vi "basic_subvi_and or search.vi"(6 "key words":string, 7 "String array input":string[](array[string])) -> (0 "or condition key words":string[](array[string]), 1 "and condition key words":string[](array[string]), 2 "index of string w/ key words":i32[](array[numeric]), 3 "output string array w/ key words":string[](array[string]))   [LabVIEW 2020, in "BasicVIs.lvlib"]
uses:
  BasicVIs.lvlib
panel:
  out "finished whole string?":bool
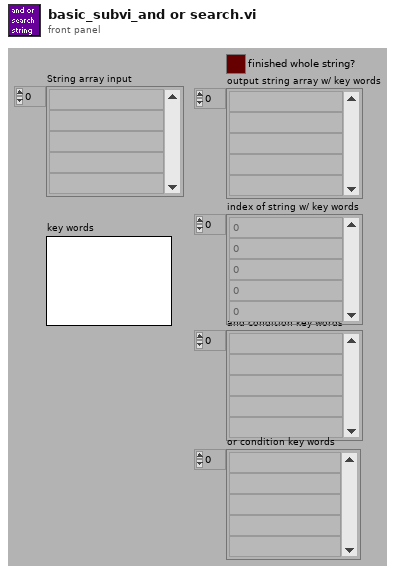
[diagram p1: front panel]
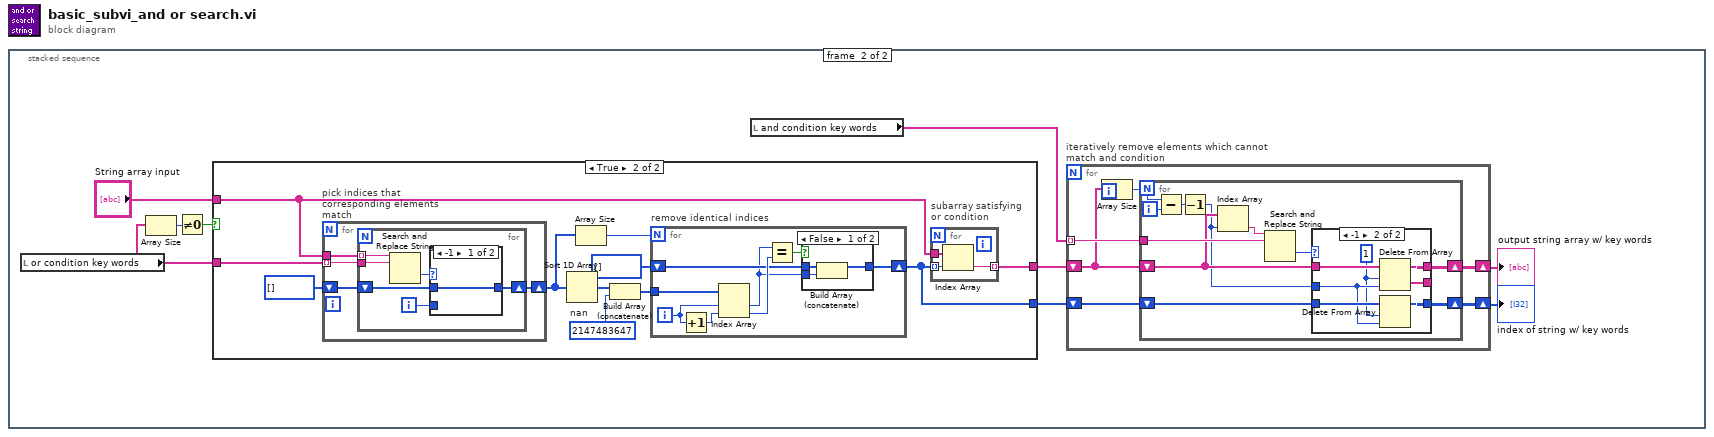
[diagram p0: block diagram]
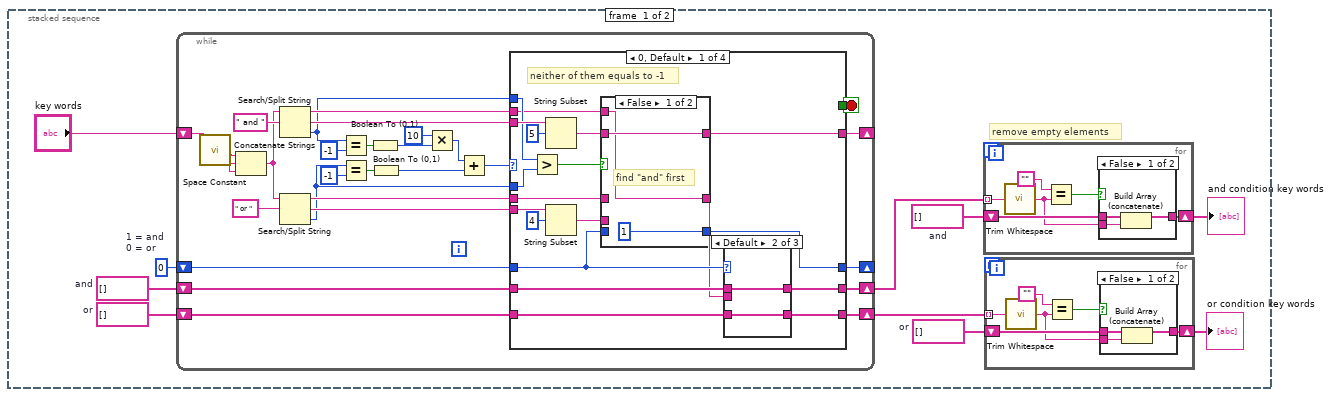
[diagram p2: hidden frame]
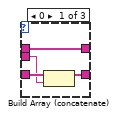
[diagram p5: hidden frame]
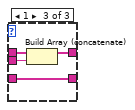
[diagram p6: hidden frame]
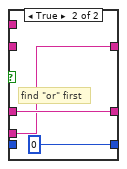
[diagram p7: hidden frame]
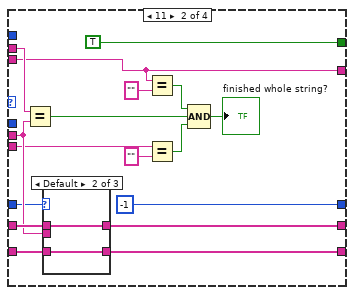
[diagram p8: hidden frame]
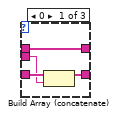
[diagram p9: hidden frame]
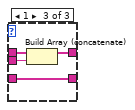
[diagram p10: hidden frame]
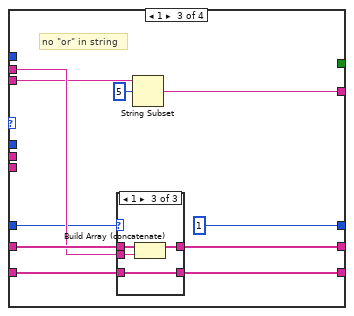
[diagram p11: hidden frame]
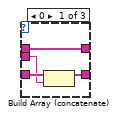
[diagram p12: hidden frame]
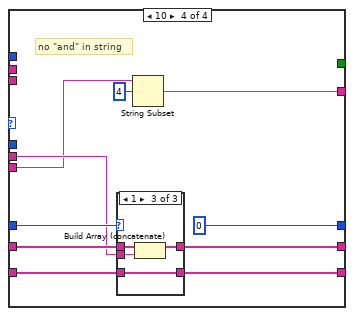
[diagram p14: hidden frame]
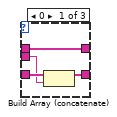
[diagram p15: hidden frame]
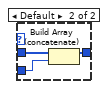
[diagram p19: hidden frame]
diagram:
  n1 = stacked-sequence {
    frame #0 {
      w6 = string[] []  # or
      w5 = string[] []  # and
      w3 = 0  # 1 = and 0 = or
      w2 = string[] []  # or
      w1 = string[] []  # and
      # "remove empty elements"
      n2 = while {
        shift-right: [w31] -> _
        shift-left: "key words" -> [w33]
        shift-right: [w39] -> w4
        shift-left: w1 -> [w41]
        shift-right: [w38] -> w7
        shift-left: w2 -> [w40]
        shift-right: [w42] -> _
        shift-left: w3 -> [w43]
        stop <- w35 stop-if-true
        n3 = call <vilib>:"Space Constant.vi"() -> ("String"=w34:string)
        n4 = Concatenate Strings(w34, w33, w34) -> (w32:string)
        n5 = Search/Split String(string=w32, search string/char (-)=" and ") -> (substring before match=w51:string, match + rest of string=w56:string, offset of match=w36:i32)  [unwired: 1 in]
        n6 = Search/Split String(string=w32, search string/char (-)=" or ") -> (substring before match=w52:string, match + rest of string=w53:string, offset of match=w44:i32)  [unwired: 1 in]
        n7 = Equal?(x=w36, y=-1) -> (x = y?=w50:bool)
        n8 = Equal?(x=w44, y=-1) -> (x = y?=w47:bool)
        n9 = Boolean To (0,1)(Boolean=w50) -> (0, 1=w49:i16)
        n10 = Boolean To (0,1)(Boolean=w47) -> (0, 1=w45:i16)
        n11 = Multiply(x=i16 10, y=w49) -> (x*y=w46:i16)
        n12 = Add(x=w46, y=w45) -> (x+y=w37:i16)
        n13 = case shown="0, Default" w37 {
          tunnel: w56 -> [w77 w100 w123 _]
          tunnel: w53 -> [w76 w98 _ w143]
          tunnel: w52 -> [w70 w103 _ w144]
          tunnel: w51 -> [w68 w108 w125 _]
          tunnel: [_ TRUE _ _] -> w35
          tunnel: w44 -> [w75 _ _ _]
          tunnel: w36 -> [w74 _ _ _]
          tunnel: [w69 w100 w122 w142] -> w31
          tunnel: w43 -> [w66 w102 w124 w145]
          tunnel: [w67 -1 ("1 = and\n0 = or") 1 ("1 = and\n0 = or") 0 ("1 = and\n0 = or")] -> w42
          tunnel: w41 -> [w65 w107 w127 w147]
          tunnel: w40 -> [w64 w106 w126 w146]
          tunnel: [w63 w104 w128 w148] -> w39
          tunnel: [w62 w105 w129 w149] -> w38
          frame 0, Default {
            # "neither of them equals to -1"
            n14 = Greater?(x=w74, y=w75) -> (0:w73:bool)
            n15 = String Subset(string=w77, offset (0)=5 ("length (rest)")) -> (substring=w71:string)  [unwired: 1 in]
            n16 = String Subset(string=w76, offset (0)=4 ("length (rest)")) -> (substring=w72:string)  [unwired: 1 in]
            n17 = case shown="False" w73 {
              tunnel: w72 -> [_ w91]
              tunnel: w71 -> [w89 _]
              tunnel: w70 -> [_ w92]
              tunnel: [w89 w91] -> w69
              tunnel: w68 -> [w88 _]
              tunnel: w66 -> [_ _]
              tunnel: [1 ("1 = and\n0 = or") 0 ("1 = and\n0 = or")] -> w67
              tunnel: [w88 w92] -> w61
              frame False {
                # "find \"and\" first"
              }
              frame True {
                # "find \"or\" first"
              }
            }
            n18 = case shown="Default" w66 {
              tunnel: w65 -> [w78 w83 w85]
              tunnel: w64 -> [w81 w82 w87]
              tunnel: [w78 w83 w86] -> w63
              tunnel: [w80 w82 w87] -> w62
              tunnel: w61 -> [w79 _ w84]
              frame 0 {
                n19 = Build Array (concatenate)(w81, w79) -> (w80:string[])
              }
              frame Default {
              }
              frame 1 {
                n20 = Build Array (concatenate)(w85, w84) -> (w86:string[])
              }
            }
          }
          frame 11 {
            n21 = Equal?(x=w108, y=w103) -> (x = y?=w96:bool)
            n22 = case shown="Default" w102 {
              tunnel: w107 -> [w111 w116 w118]
              tunnel: w106 -> [w114 w115 w120]
              tunnel: [w111 w116 w119] -> w104
              tunnel: [w113 w115 w120] -> w105
              tunnel: w103 -> [w112 _ w117]
              frame 0 {
                n23 = Build Array (concatenate)(w114, w112) -> (w113:string[])
              }
              frame Default {
              }
              frame 1 {
                n24 = Build Array (concatenate)(w118, w117) -> (w119:string[])
              }
            }
            n25 = Equal?(x=w100, y="" ("key words of filter")) -> (x = y?=w97:bool)
            n26 = Equal?(x=w98, y="" ("key words of filter")) -> (x = y?=w95:bool)
            n27 = Compound Arithmetic op=AND(w97, w96, w95) -> (→"finished whole string?":bool)
          }
          frame 1 {
            # "no \"or\" in string"
            n28 = case shown="1" w124 {
              tunnel: w127 -> [w131 w136 w138]
              tunnel: w126 -> [w134 w135 w140]
              tunnel: [w131 w136 w139] -> w128
              tunnel: [w133 w135 w140] -> w129
              tunnel: w125 -> [w132 _ w137]
              frame 0 {
                n29 = Build Array (concatenate)(w134, w132) -> (w133:string[])
              }
              frame Default {
              }
              frame 1 {
                n30 = Build Array (concatenate)(w138, w137) -> (w139:string[])
              }
            }
            n31 = String Subset(string=w123, offset (0)=5 ("length (rest)")) -> (substring=w122:string)  [unwired: 1 in]
          }
          frame 10 {
            # "no \"and\" in string"
            n32 = case shown="1" w145 {
              tunnel: w147 -> [w151 w156 w158]
              tunnel: w146 -> [w154 w155 w160]
              tunnel: [w151 w156 w159] -> w148
              tunnel: [w153 w155 w160] -> w149
              tunnel: w144 -> [w152 _ w157]
              frame 0 {
                n33 = Build Array (concatenate)(w154, w152) -> (w153:string[])
              }
              frame Default {
              }
              frame 1 {
                n34 = Build Array (concatenate)(w158, w157) -> (w159:string[])
              }
            }
            n35 = String Subset(string=w143, offset (0)=4 ("length (rest)")) -> (substring=w142:string)  [unwired: 1 in]
          }
        }
      }
      n36 = for {
        tunnel: w4 -> [w26] mode=indexing
        shift-right: [w22] -> w10
        shift-left: w5 -> [w23]
        n37 = call <vilib>:"Trim Whitespace.vi"("string"=w26) -> ("trimmed string"=w21:string)  [unwired: 1 in]
        n38 = Equal?(x="", y=w21) -> (x = y?=w24:bool)
        n39 = case shown="False" w24 {
          tunnel: w23 -> [w29 w30]
          tunnel: [w27 w30] -> w22
          tunnel: w21 -> [w28 _]
          frame False {
            n40 = Build Array (concatenate)(w29, w28) -> (w27:string[])
          }
          frame True {
          }
        }
      }
      "and condition key words" <- w10
      n41 = for {
        tunnel: w7 -> [w16] mode=indexing
        shift-right: [w12] -> w9
        shift-left: w6 -> [w13]
        n42 = call <vilib>:"Trim Whitespace.vi"("string"=w16) -> ("trimmed string"=w11:string)  [unwired: 1 in]
        n43 = Equal?(x="", y=w11) -> (x = y?=w14:bool)
        n44 = case shown="False" w14 {
          tunnel: w13 -> [w19 w20]
          tunnel: [w17 w20] -> w12
          tunnel: w11 -> [w18 _]
          frame False {
            n45 = Build Array (concatenate)(w19, w18) -> (w17:string[])
          }
          frame True {
          }
        }
      }
      "or condition key words" <- w9
    }
    frame #1 {
      n46 = local read "or condition key words"() -> (w163:string[])
      n47 = Array Size(array=w163) -> (size(s)=w162:i32)
      n48 = Not Equal To 0?(x=w162) -> (x != 0?=w161:bool)
      n49 = case shown="True" w161 {
        tunnel: [w170 w183] -> w168
        tunnel: [w171 w182] -> w167
        tunnel: "String array input" -> [w171 w181]
        tunnel: w163 -> [_ w173]
        frame False {
          n50 = for {
            tunnel: w171 -> [_] mode=indexing
            tunnel: [w172] -> w170 mode=indexing
            i -> [w172]
          }
        }
        frame True {
          w178 = 2147483647  # nan
          n51 = for "pick indices that corresponding elements match" {
            tunnel: w173 -> [w202] mode=indexing
            tunnel: w181 -> [w201]
            shift-right: [w200] -> w175
            shift-left: i32[] [] -> [w199]
            n52 = for {
              tunnel: w202 -> [w204]
              tunnel: w201 -> [w205] mode=indexing
              shift-right: [w207] -> w200
              shift-left: w199 -> [w206]
              i -> [w208]
              n53 = Search and Replace String(input string=w205, search string=w204) -> (offset past replacement=w203:i32)  [unwired: 6 in, 3 out]
              n54 = case shown="-1" w203 {
                tunnel: w208 -> [_ w211]
                tunnel: [w209 w210] -> w207
                tunnel: w206 -> [w209 w212]
                frame -1 {
                }
                frame Default {
                  n55 = Build Array (concatenate)(w212, w211) -> (w210:i32[])
                }
              }
            }
          }
          n56 = Sort 1D Array(array=w175) -> (sorted array=w176:i32[])
          n57 = Array Size(array=w175) -> (size(s)=w177:i32)
          n58 = Build Array (concatenate)(w176, w178) -> (w179:i32[])
          n59 = for "remove identical indices" {
            N: w177 -> [_]
            tunnel: w179 -> [w194]
            shift-right: [w188] -> w183
            shift-left: i32[] [] -> [w189]
            i -> [w193]
            n60 = Increment(x=w193) -> (x+1=w192:i32)
            n61 = Index Array(array=w194, index #1=w193, index #2=w192) -> (element #1=w187:i32, element #2=w191:i32)
            n62 = Equal?(x=w187, y=w191) -> (x = y?=w190:bool)
            n63 = case shown="False" w190 {
              tunnel: w189 -> [w197 w198]
              tunnel: [w195 w198] -> w188
              tunnel: w187 -> [w196 _]
              frame False {
                n64 = Build Array (concatenate)(w197, w196) -> (w195:i32[])
              }
              frame True {
              }
            }
          }
          n65 = for "subarray satisfying\nor condition" {
            tunnel: w183 -> [w185] mode=indexing
            tunnel: w181 -> [w186]
            tunnel: [w184] -> w182 mode=indexing
            n66 = Index Array(array=w186, index=w185) -> (element=w184:string)
          }
        }
      }
      n67 = local read "and condition key words"() -> (w169:string[])
      n68 = for "iteratively remove elements which cannot match and condition" {
        tunnel: w169 -> [w218] mode=indexing
        shift-right: [w214] -> w164
        shift-left: w167 -> [w215]
        shift-right: [w213] -> w165
        shift-left: w168 -> [w217]
        n69 = Array Size(array=w215) -> (size(s)=w216:i32)
        n70 = for {
          N: w216 -> [w228]
          tunnel: w218 -> [w229]
          shift-right: [w223] -> w214
          shift-left: w215 -> [w224]
          shift-right: [w221] -> w213
          shift-left: w217 -> [w222]
          i -> [w227]
          n71 = Subtract(x=w228, y=w227) -> (x-y=w226:i32)
          n72 = Decrement(x=w226) -> (x-1=w220:i32)
          n73 = Index Array(array=w224, index=w220) -> (element=w225:string)
          n74 = Search and Replace String(input string=w225, search string=w229) -> (offset past replacement=w219:i32)  [unwired: 6 in, 3 out]
          n75 = case shown="-1" w219 {
            tunnel: w224 -> [w231 w238]
            tunnel: [w231 w237] -> w223
            tunnel: w222 -> [w230 w236]
            tunnel: [w230 w235] -> w221
            tunnel: w220 -> [_ w234]
            tunnel: [_ w232] -> _
            frame Default {
            }
            frame -1 {
              w233 = 1 ("length")
              n76 = Delete From Array(array=w238, length=w233, index=w234) -> (deleted portion=w232:string[], array with subset deleted=w237:string[])
              n77 = Delete From Array(array=w236, length=w233, index=w234) -> (array with subset deleted=w235:i32[])  [unwired: 1 out]
            }
          }
        }
      }
      "index of string w/ key words" <- w165
      "output string array w/ key words" <- w164
    }
  }
